vi "2.1.vi"() -> ()   [LabVIEW 2017]
panel:
  in  "停止":bool
  in  "比例系数":dbl
  in  "相乘":bool
  in  "数值":dbl
  # "任务一"
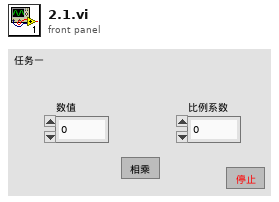
[diagram p1: front panel]
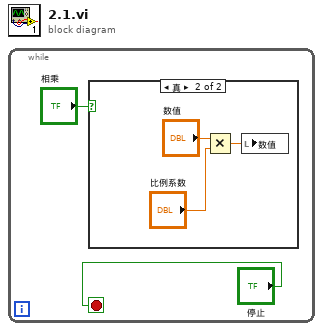
[diagram p0: block diagram]
diagram:
  n1 = while {
    stop <- "停止" stop-if-true
    n2 = case shown="真" "相乘" {
      frame False {
      }
      frame True {
        n3 = Multiply(x="数值", y="比例系数") -> (x*y=w3:dbl)
        n4 = local write "数值"(w3) -> ()
      }
    }
  }
